vi "Read String.vi"(8 "error in (no error)":errorcluster, 11 "UDP in":refnum<class "UDP.lvclass">) -> (0 "error out":errorcluster, 1 "Bytes Read":i32, 2 "String Read":string, 3 "UDP out":refnum<class "UDP.lvclass">)   [LabVIEW 2024, in "UDP.lvclass"]
doc: "UPS.lvclass:Read String.vi\n\nThis is the Read String VI forthe UDP class.\n\nInstrument Communication Module Version 1.0\nJanuary, 2017 Original Code Consulting David Thomson\n www.originalcode.com"
uses:
  UDP.lvclass
  UDP.lvclass/UDP.ctl
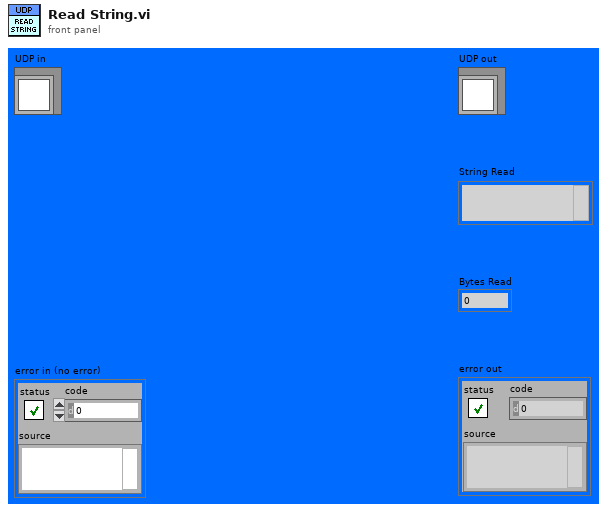
[diagram p1: front panel]
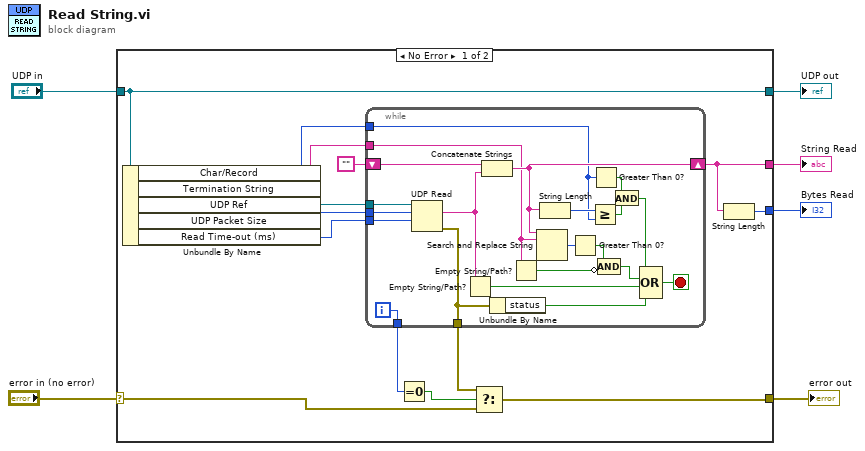
[diagram p0: block diagram]
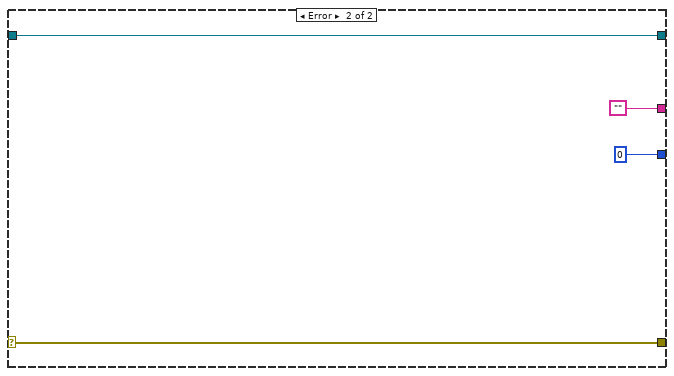
[diagram p2: hidden frame]
diagram:
  n1 = case shown="No Error" "error in (no error)" {
    selector: "error in (no error)" -> [w9 w45]
    tunnel: [w10 w45] -> w5
    tunnel: [w12 w44] -> w4
    tunnel: "UDP in" -> [w12 w44]
    tunnel: [w18 ""] -> w2
    tunnel: [w19 0 ("Bytes Read")] -> w1
    frame No Error {
      n2 = Unbundle By Name(w12) -> ("Char/Record"=w13:i32, "Termination String"=w14:string, "UDP Ref"=w17:refnum<k16>, "UDP Packet Size"=w16:i32, "Read Time-out (ms)"=w15:i32)
      n3 = while {
        tunnel: w17 -> [w41]
        tunnel: w16 -> [w40]
        shift-right: [w26] -> w18
        shift-left: "" -> [w36]
        tunnel: w15 -> [w34]
        tunnel: w14 -> [w24]
        tunnel: w13 -> [w23]
        tunnel: [w22] -> w11
        tunnel: [w21] -> w8
        i -> [w21]
        stop <- w37 stop-if-true
        n4 = UDP Read(connection ID=w41, max size (548)=w40, timeout ms (25000)=w34) -> (data out=w35:string, error out=w22:errorcluster)  [unwired: 1 in, 3 out]
        n5 = Empty String/Path?(string/path=w35) -> (empty?=w39:bool)
        n6 = Concatenate Strings(w36, w35) -> (w26:string)
        n7 = Unbundle By Name(w22) -> ("status"=w38:bool)
        n8 = Empty String/Path?(string/path=w24) -> (empty?=w29:bool)
        n9 = Search and Replace String(input string=w26, search string=w24) -> (number of replacements=w28:i32)  [unwired: 1 in, 8 out]
        n10 = String Length(string=w26) -> (length=w31:i32)
        n11 = Greater Than 0?(x=w28) -> (x > 0?=w27:bool)
        n12 = Greater Or Equal?(x=w31, y=w23) -> (x >= y?=w32:bool)
        n13 = Greater Than 0?(x=w23) -> (x > 0?=w33:bool)
        n14 = Compound Arithmetic op=AND(w27, invert w29) -> (w25:bool)
        n15 = And(x=w33, y=w32) -> (x .and. y?=w30:bool)
        n16 = Compound Arithmetic op=OR(w30, w25, w39, w38) -> (w37:bool)
      }
      n17 = Equal To 0?(x=w8) -> (x = 0?=w7:bool)
      n18 = Select(t=w11, s=w7, f=w9) -> (s? t:f=w10:errorcluster)
      n19 = String Length(string=w18) -> (length=w19:i32)
    }
    frame Error {
    }
  }
  "error out" <- w5
  "UDP out" <- w4
  "Bytes Read" <- w1
  "String Read" <- w2
